vi "Exposure Noise Synthesis Test.vi"() -> ()   [LabVIEW 2015]
uses:
  Calibration VIs/Inverse Filter VIs/InvFilt-Params.ctl
  Utility VIs/Math VIs/FFT x(t) to dB,Degrees (1D).vi
  Utility VIs/Math VIs/LinSpace (x0-dx-npts).vi
panel:
  in  "Precompensate":bool
  out "XY Graph":T1(graph)
  in  "InvFilt Params":T2={"Min Frequency (Hz)"=1000.0, "Max Frequency (Hz)"=100000.0, "Length (points)"=301, "Sampling rate (Hz)"=100000.0, "Delay (ms)"=1.5, "Linear phase"=FALSE}
  in  "Calibration file":path=path "U:/Shared/Hancock/z.Data/Calibrations/Example Calibrations/RightPrimary.calib"
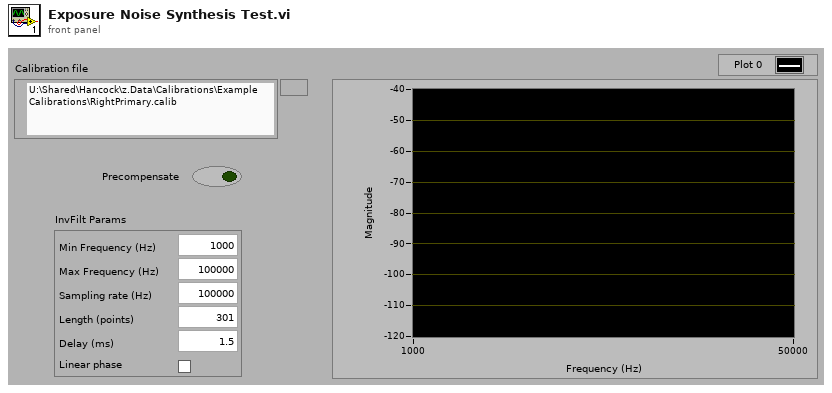
[diagram p1: front panel]
types:
  T1 = cluster{"Array":dbl[], "+Freq. Mag of FFT (dB rms)":dbl[]}[]
  T2 = typedef "InvFilt-Params.ctl" = cluster{"Min Frequency (Hz)":dbl, "Max Frequency (Hz)":dbl, "Length (points)":i32, "Sampling rate (Hz)":dbl, "Delay (ms)":dbl, "Linear phase":bool}
  T3 = cluster{"Array":dbl[], "+Freq. Mag of FFT (dB rms)":dbl[]}
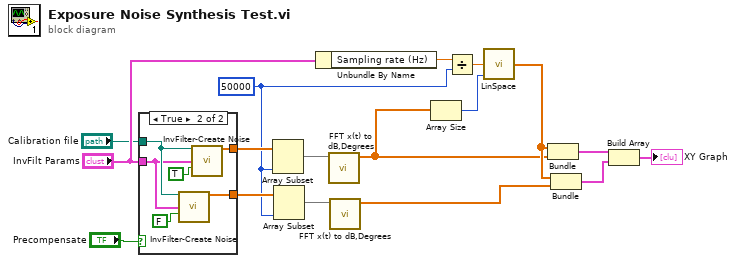
[diagram p0: block diagram]
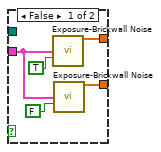
[diagram p2: hidden frame]
diagram:
  w3 = 50000 ("length")
  n1 = case shown="True" "Precompensate" {
    tunnel: "InvFilt Params" -> [w21 w24]
    tunnel: [w19 w28] -> w10
    tunnel: [w18 w26] -> w9
    tunnel: "Calibration file" -> [_ w25]
    frame False {
      n2 = call "Exposure-Brickwall Noise.vi"("InvFilt Params"=w21, "Brickwall (T)"=TRUE) -> ("Noise"=w19:dbl[])  [unwired: 11 in, 2 out]
      n3 = call "Exposure-Brickwall Noise.vi"("InvFilt Params"=w21, "Brickwall (T)"=FALSE) -> ("Noise"=w18:dbl[])  [unwired: 11 in, 2 out]
    }
    frame True {
      n4 = call "InvFilter-Create Noise.vi"("Calibration File"=w25, "InvFilt Params"=w24, "Brickwall (T)"=FALSE) -> ("InvFilter Noise"=w26:dbl[])  [unwired: 9 in, 3 out]
      n5 = call "InvFilter-Create Noise.vi"("Calibration File"=w25, "InvFilt Params"=w24, "Brickwall (T)"=TRUE) -> ("InvFilter Noise"=w28:dbl[])  [unwired: 9 in, 3 out]
    }
  }
  n6 = Array Subset(array=w10, length=w3) -> (w8:dbl[])  [unwired: 1 in]
  n7 = Array Subset(array=w9, length=w3) -> (w6:dbl[])  [unwired: 1 in]
  n8 = Unbundle By Name("InvFilt Params") -> ("Sampling rate (Hz)"=w17:dbl)
  n9 = call-poly "FFT x(t) to dB,Degrees.vi"("X"=w8) -> ("+Freq. Mag of FFT (dB rms)"=w7:dbl[])  [unwired: 8 in, 2 out]
  n10 = call-poly "FFT x(t) to dB,Degrees.vi"("X"=w6) -> ("+Freq. Mag of FFT (dB rms)"=w5:dbl[])  [unwired: 8 in, 2 out]
  n11 = Array Size(array=w7) -> (size(s)=w4:i32)
  n12 = Divide(x=w17, y=w3) -> (x/y=w16:dbl)
  n13 = call-poly "LinSpace.vi"("npts"=w4, "dx"=w16) -> ("Array"=w14:dbl[])  [unwired: 2 in, 1 out]
  n14 = Bundle("Array"=w14, "+Freq. Mag of FFT (dB rms)"=w7) -> (w13:T3)  [unwired: 1 in]
  n15 = Bundle("Array"=w14, "+Freq. Mag of FFT (dB rms)"=w5) -> (w12:T3)  [unwired: 1 in]
  n16 = Build Array(w13, w12) -> (→"XY Graph":T1)
